vi "Calculator-test_harness.vi"(11 "test case ID":string) -> (3 "result":bool)   [LabVIEW 2018]
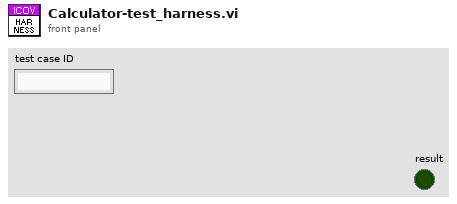
[diagram p1: front panel]
types:
  T1 = typedef "Operation--enum.ctl" = enum16{"Add (X + Y)", "Subtract (X - Y)", "Multiply (X * Y)", "Divide (X / Y)"}
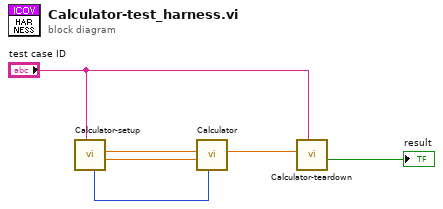
[diagram p0: block diagram]
diagram:
  n1 = call "Calculator-setup.vi"("test case ID"="test case ID") -> ("Y"=w3:dbl, "X"=w4:dbl, "Operation"=w2:T1)  [unwired: 8 in]
  n2 = call "Calculator.vi"("Operation"=w2, "Y"=w3, "X"=w4) -> ("Result"=w1:dbl)  [unwired: 8 in]
  n3 = call "Calculator-teardown.vi"("test case ID"="test case ID", "Actual result"=w1) -> ("result"=→"result":bool)  [unwired: 9 in]
